vi "Problem1.5.vi"() -> ()   [LabVIEW 2019]
panel:
  in  "Reset":bool
  in  "Set":bool
  out "Output Negation":bool
  out "Output":bool
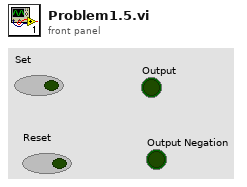
[diagram p1: front panel]
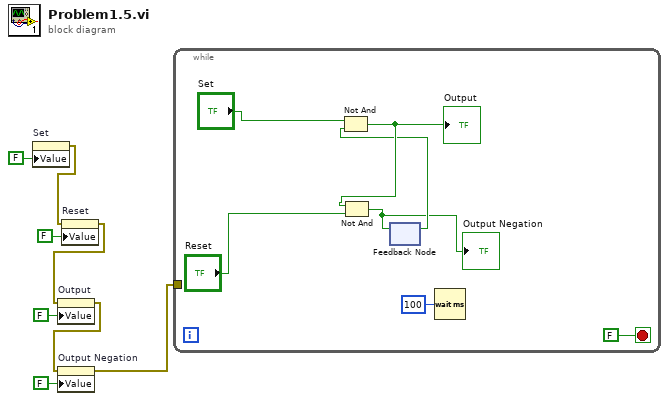
[diagram p0: block diagram]
diagram:
  n1 = property on="Set" class="Bool (strict)"("Value"=FALSE ("Set")) -> (error out=w4:errorcluster)  [unwired: 2 in, 1 out]
  n2 = property on="Reset" class="Bool (strict)"(error in=w4, "Value"=FALSE ("Reset")) -> (error out=w3:errorcluster)  [unwired: 1 in, 1 out]
  n3 = property on="Output" class="Bool (strict)"(error in=w3, "Value"=FALSE ("Output")) -> (error out=w2:errorcluster)  [unwired: 1 in, 1 out]
  n4 = property on="Output Negation" class="Bool (strict)"(error in=w2, "Value"=FALSE ("Output Negation")) -> (error out=w1:errorcluster)  [unwired: 1 in, 1 out]
  n5 = while {
    tunnel: w1 -> [_]
    stop <- FALSE stop-if-true
    n6 = feedback #1() -> (w10:bool)  [unwired: 1 in]
    n7 = Not And(1:w10, 2:"Set") -> (0:w11:bool)
    "Output" <- w11
    n8 = Not And(1:"Reset", 2:w11) -> (0:w9:bool)
    "Output Negation" <- w9
    n9 = feedback-in #1(w9) -> ()
    n10 = Wait (ms)(milliseconds to wait=u32 100) -> ()  [unwired: 1 out]
  }
